vi "Configure Channel.vi"(0 "VISA resource name":refnum<visa-resource-name>, 1 "Enable Channel (True)":bool=TRUE, 5 "Channel (0: Channel 1)":i32(ring) items=["Channel 1", "Channel 2", "Channel 3", "Channel 4", "Math", "Reference A", "Reference B", "Reference C", "Reference D"], 7 "Vertical Coupling (1: DC)":i32(ring)=1 items=["AC", "DC", "Ground"], 9 "Probe Attenuation (10: 10X)":i32(ring)=10 items=["1"=1, "10"=10, "20"=20, "50"=50, "100"=100, "500"=500, "1000"=1000], 11 "error in (no error)":errorcluster, 12 "Vertical Range (10.0 V/div)":dbl=10.0, 13 "Vertical Offset (0.0 divs)":dbl, 14 "Bandwidth (0: MAX Bandwidth)":i32(ring) items=["MAX Bandwidth", "Unlimited"]) -> (4 "VISA resource name out":refnum<visa-resource-name>, 15 "error out":errorcluster)   [LabVIEW 2017, in "Tektronix TDS 200 1000 2000 Series.lvlib"]
doc: "Configures the common properties of the oscilloscope's vertical subsystem for the specified channel. Call this VI for each channel you want to enable to acquire waveforms.\n\n<b>Note(s):</b>\nThe channel settings will not be applied if the channel is not enabled."
uses:
  Tektronix TDS 200 1000 2000 Series.lvlib
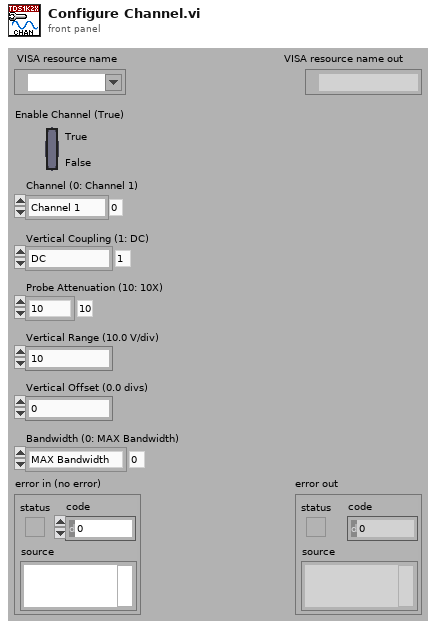
[diagram p1: front panel]
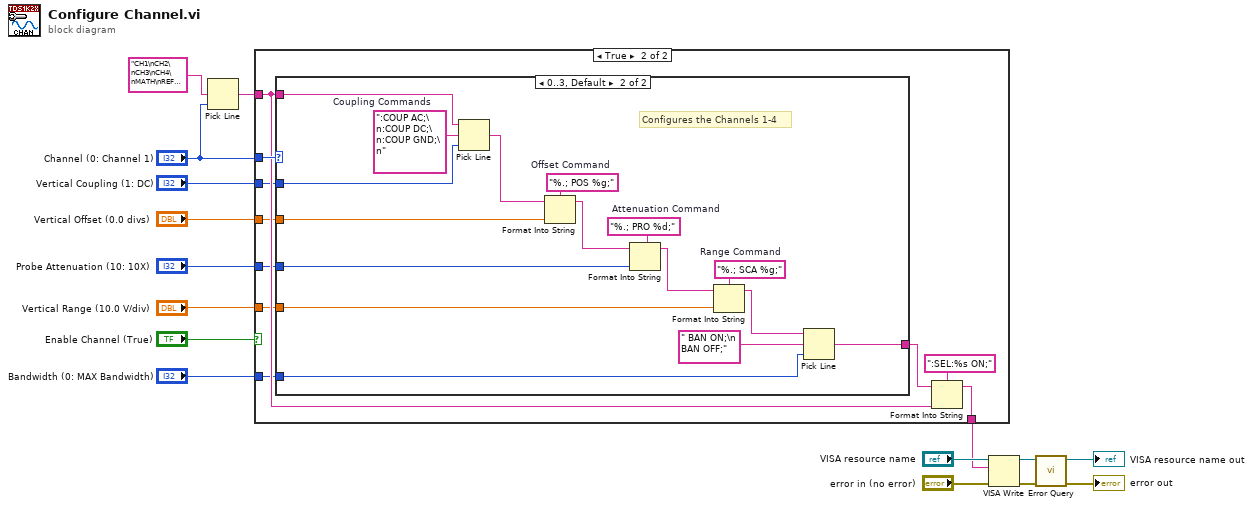
[diagram p0: block diagram]
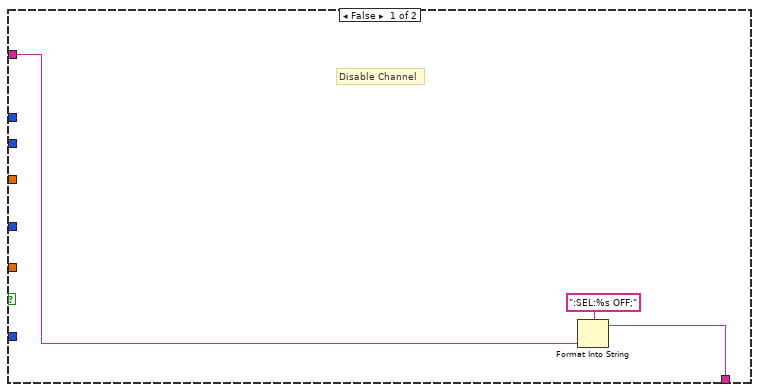
[diagram p2: hidden frame]
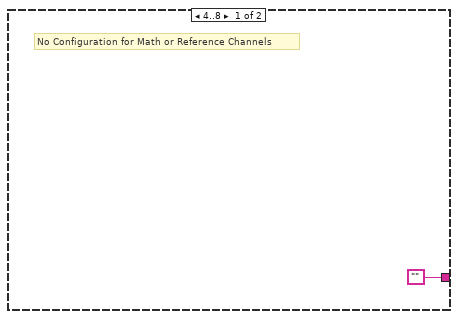
[diagram p3: hidden frame]
diagram:
  n1 = Pick Line(multi-line string="CH1\nCH2\nCH3\nCH4\nMATH\nREFA\nREFB\nREFC\nREFD", line index="Channel (0: Channel 1)") -> (output string=w6:string)  [unwired: 1 out]
  n2 = case shown="True" "Enable Channel (True)" {
    tunnel: [w18 w28] -> w10
    tunnel: w6 -> [w17 w25]
    tunnel: "Channel (0: Channel 1)" -> [_ w26]
    tunnel: "Vertical Coupling (1: DC)" -> [_ w24]
    tunnel: "Vertical Offset (0.0 divs)" -> [_ w23]
    tunnel: "Probe Attenuation (10: 10X)" -> [_ w22]
    tunnel: "Vertical Range (10.0 V/div)" -> [_ w21]
    tunnel: "Bandwidth (0: MAX Bandwidth)" -> [_ w20]
    frame False {
      # "Disable Channel"
      n3 = Format Into String(format string=":SEL:%s OFF;", w17) -> (resulting string=w18:string)  [unwired: 2 in, 1 out]
    }
    frame True {
      n4 = case shown="0..3, Default" w26 {
        tunnel: ["" w40] -> w27
        tunnel: w25 -> [_ w41]
        tunnel: w24 -> [_ w35]
        tunnel: w23 -> [_ w34]
        tunnel: w22 -> [_ w33]
        tunnel: w21 -> [_ w32]
        tunnel: w20 -> [_ w31]
        frame 4..8 {
          # "No Configuration for Math or Reference Channels"
        }
        frame 0..3, Default {
          w43 = "%.; PRO %d;"  # Attenuation Command
          w44 = "%.; SCA %g;"  # Range Command
          w45 = "%.; POS %g;"  # Offset Command
          w46 = ":COUP AC;\n:COUP DC;\n:COUP GND;\n"  # Coupling Commands
          # "Configures the Channels 1-4"
          n5 = Pick Line(string ("")=w41, multi-line string=w46, line index=w35) -> (output string=w42:string)
          n6 = Format Into String(format string=w45, initial string=w42, w34) -> (resulting string=w38:string)  [unwired: 1 in, 1 out]
          n7 = Format Into String(format string=w43, initial string=w38, w33) -> (resulting string=w37:string)  [unwired: 1 in, 1 out]
          n8 = Format Into String(format string=w44, initial string=w37, w32) -> (resulting string=w36:string)  [unwired: 1 in, 1 out]
          n9 = Pick Line(string ("")=w36, multi-line string=" BAN ON;\n BAN OFF;", line index=w31) -> (output string=w40:string)
        }
      }
      n10 = Format Into String(format string=":SEL:%s ON;", initial string=w27, w25) -> (resulting string=w28:string)  [unwired: 1 in, 1 out]
    }
  }
  n11 = VISA Write(VISA resource name="VISA resource name", write buffer=w10, error in (no error)="error in (no error)") -> (VISA resource name out=w12:refnum<visa-resource-name>, error out=w11:errorcluster)  [unwired: 1 out]
  n12 = call "Error Query.vi"("error in (no error)"=w11, "VISA resource name"=w12) -> ("error out"=→"error out":errorcluster, "VISA resource name out"=→"VISA resource name out":refnum<visa-resource-name>)  [unwired: 8 out]
